vi "bytea sandbox.vi"() -> ()   [LabVIEW 2019, in "LV-Data.PGSQL.lvclass"]
uses:
  LV-Data.PGSQL.lvclass
  <vilib>/numeric/Random Number (Range) U64.vi
  <vilib>/numeric/sub_Random U32.vi
panel:
  in  "number?":bool
  in  "string?":bool
  in  "string":string
  out "hex string":string
  out "resulting string":string
  out "number":u64
  out "error out":errorcluster
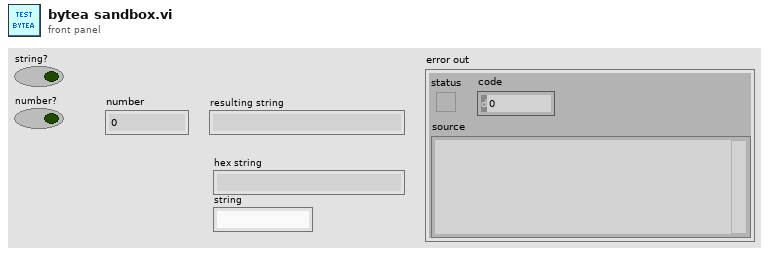
[diagram p1: front panel]
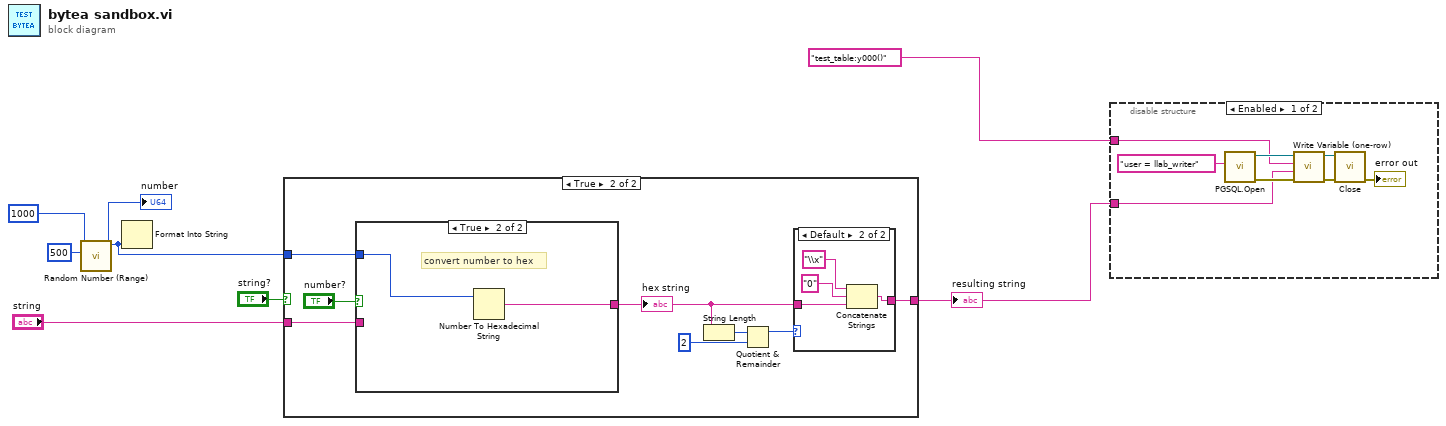
[diagram p0: block diagram]
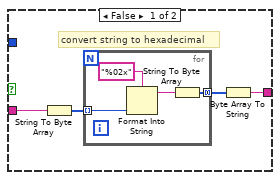
[diagram p3: hidden frame]
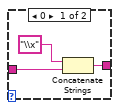
[diagram p4: hidden frame]
diagram:
  n1 = call-poly <vilib>:"Random Number (Range).vi"("lower bound (0)"=u64 500, "upper bound (100)"=u64 1000) -> ("number"=w3:u64)  [unwired: 9 in]
  "number" <- w3
  n2 = Format Into String(w3) -> ()  [unwired: 3 in, 2 out]
  n3 = case shown="True" "string?" {
    tunnel: "string" -> [w8 w13]
    tunnel: [w8 w11] -> w2
    tunnel: w3 -> [_ w10]
    frame False {
      # "let postgres convert a string to hex"
    }
    frame True {
      n4 = case shown="True" "number?" {
        tunnel: w13 -> [w18 _]
        tunnel: [w17 w26] -> w12
        tunnel: w10 -> [_ w25]
        frame False {
          # "convert string to hexadecimal"
          n5 = String To Byte Array(string=w18) -> (unsigned byte array=w20:u8[])
          n6 = for {
            tunnel: w20 -> [w24] mode=indexing
            tunnel: [w21] -> w19 mode=concatenating
            n7 = Format Into String(format string="%02x", w24) -> (resulting string=w22:string)  [unwired: 2 in, 1 out]
            n8 = String To Byte Array(string=w22) -> (unsigned byte array=w21:u8[])
          }
          n9 = Byte Array To String(unsigned byte array=w19) -> (string=w17:string)
        }
        frame True {
          # "convert number to hex"
          n10 = Number To Hexadecimal String(2:w25) -> (0:w26:string)  [unwired: 1 in]
        }
      }
      "hex string" <- w12
      n11 = String Length(string=w12) -> (length=w16:i32)
      n12 = Quotient & Remainder(x=w16, y=2) -> (x-y*floor(x/y)=w14:i32)  [unwired: 1 out]
      n13 = case shown="Default" w14 {
        tunnel: [w28 w32] -> w11
        tunnel: w12 -> [w27 w31]
        frame 0 {
          n14 = Concatenate Strings("\\x" ("string"), w27) -> (w28:string)
        }
        frame Default {
          n15 = Concatenate Strings("\\x" ("string"), "0" ("string"), w31) -> (w32:string)
        }
      }
    }
  }
  "resulting string" <- w2
  n16 = disable-structure shown="Enabled" {
    disable-tunnel: w2 -> [w35 _]
    disable-tunnel: "test_table:y000()" ("SQL") -> [w34 _]
    frame Enabled {
      n17 = call "PGSQL.Open.vi"("Connection String"="user = llab_writer") -> ("error out"=w36:errorcluster, "Data.PG out"=w39:refnum<class "LV-Data.PGSQL.lvclass">)  [unwired: 9 in]
      n18 = call "Write Variable (one-row).vi"("error in (no error)"=w36, "Data"=w35, "Paths"=w34, "Data.PG in"=w39) -> ("error out"=w37:errorcluster, "Data.PG out"=w38:refnum<class "LV-Data.PGSQL.lvclass">)  [unwired: 4 in, 2 out]
      n19 = call-dynamic "Close.vi"("error in (no error)"=w37, "Data.PG in"=w38) -> ("error out"=→"error out":errorcluster)  [unwired: 8 in, 1 out]
    }
    frame Disabled {
    }
  }
